vi "Save DAQ Configuration.vi"(8 "Error In":errorcluster, 10 "DAQ Device Settings":T1={"Analog Input Channel"="Dev1/ai0", "AImin[V]"=0, "AImax[V]"=5, "Analog Output Channel"="Dev1/ao0", "AOmin[V]"=0, "AOmax[V]"=5} {"AOmax[V]" min=-10 max=10 step=1 format="%.0g"; "AOmin[V]" min=-10 max=10 step=1 format="%.0g"; "AImax[V]" min=-10 max=10 step=1 format="%.0g"; "AImin[V]" min=-10 max=10 step=1 format="%.0g"}) -> (0 "Error Out":errorcluster)   [LabVIEW 2018]
uses:
  <vilib>/Utility/config.llb/Write Key (String).vi
  <vilib>/Utility/config.llb/Write Key (I32).vi
  <vilib>/Utility/config.llb/NI_LVConfig.lvlib
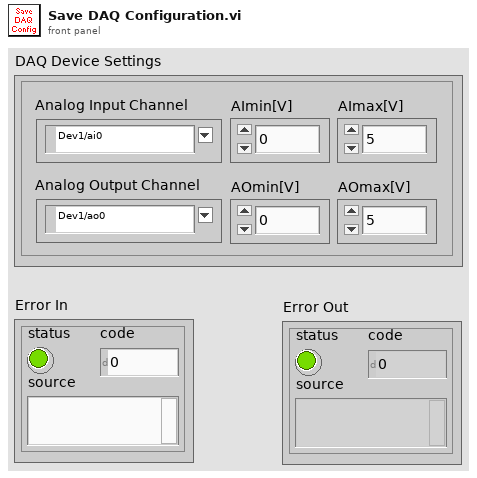
[diagram p1: front panel]
types:
  T1 = cluster{"Analog Input Channel":tag, "AImin[V]":i32, "AImax[V]":i32, "Analog Output Channel":tag, "AOmin[V]":i32, "AOmax[V]":i32}
  T2 = typedef "NI_LVConfig.lvlib/Config Data RefNum.ctl" = refnum<k1>
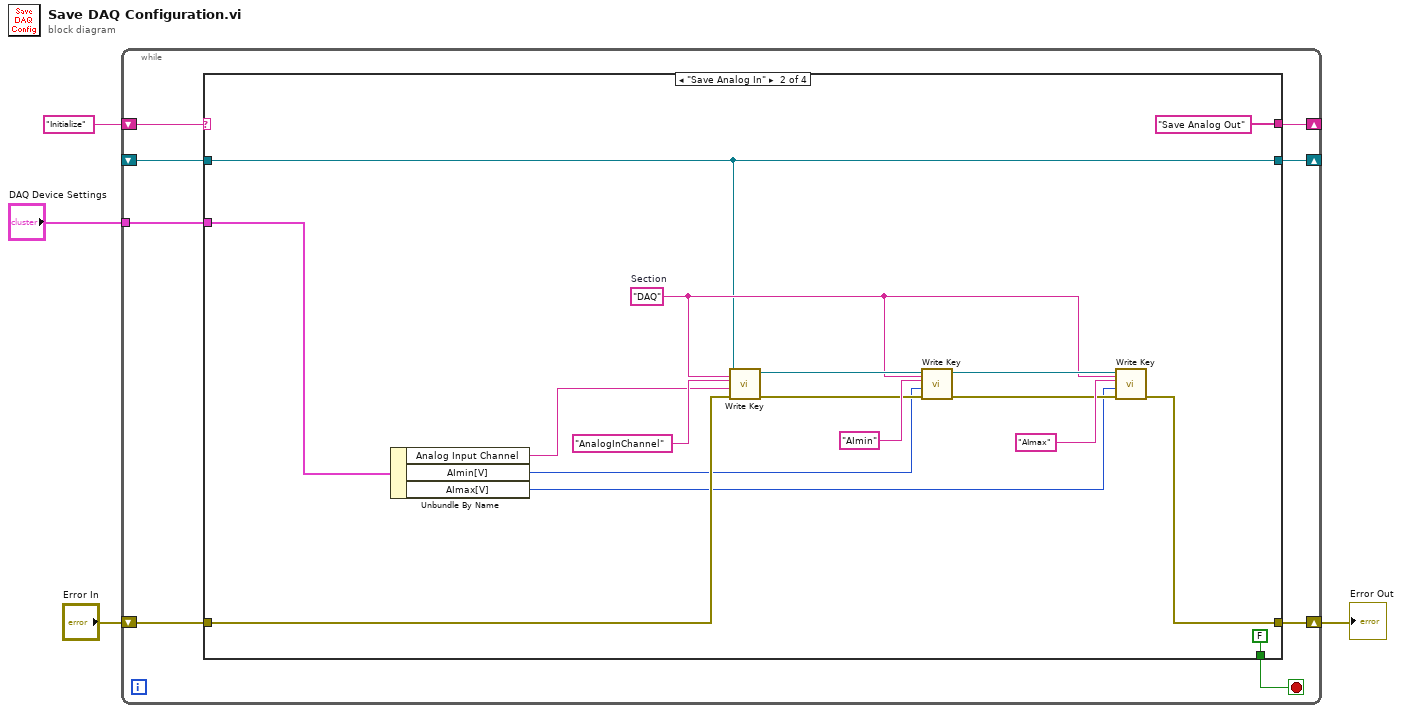
[diagram p0: block diagram]
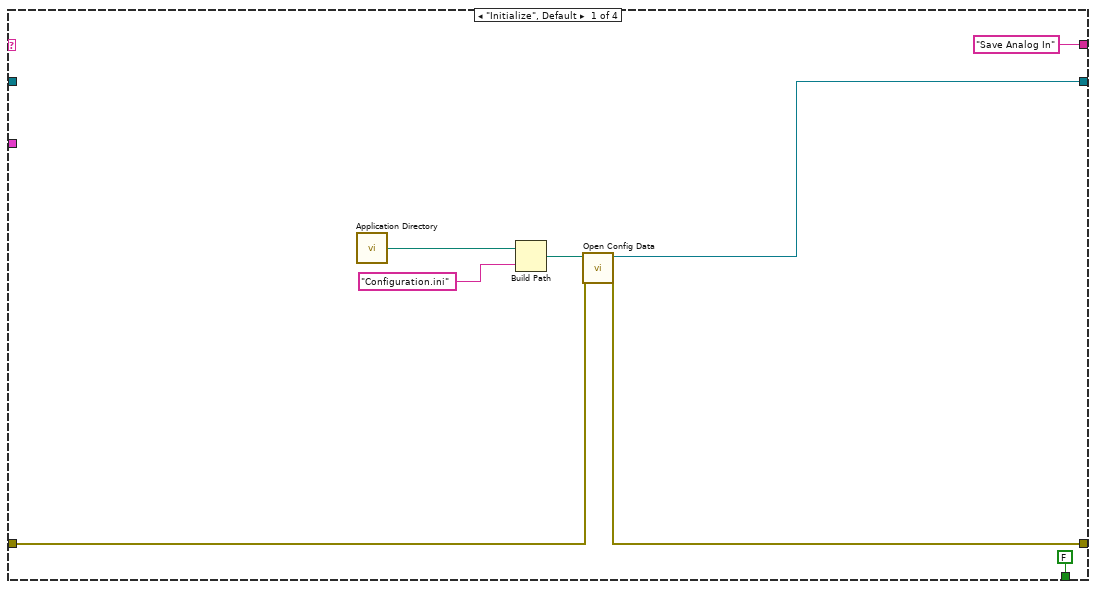
[diagram p2: hidden frame]
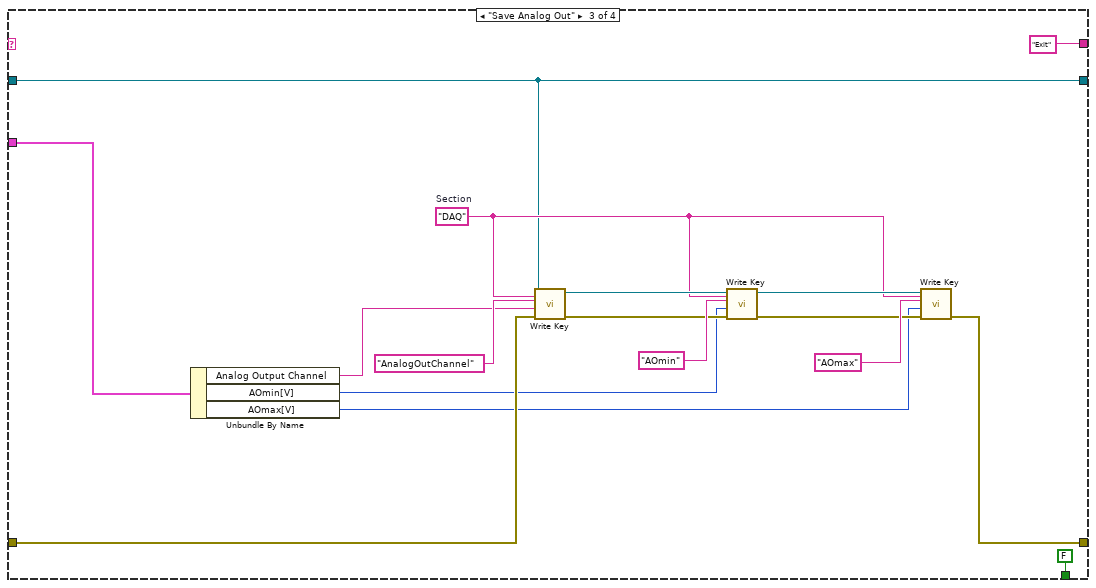
[diagram p3: hidden frame]
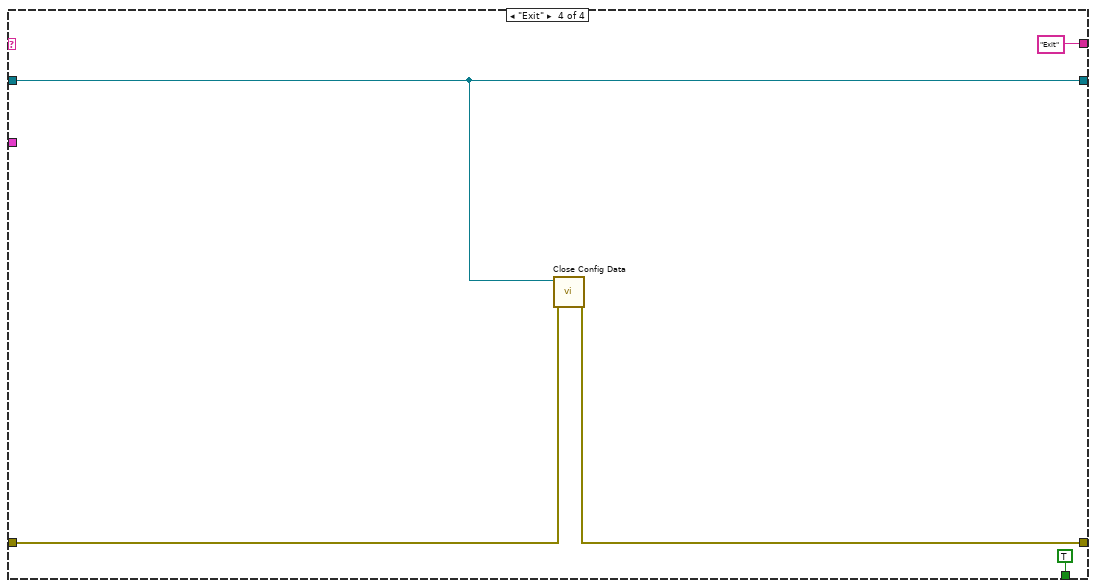
[diagram p4: hidden frame]
diagram:
  n1 = while {
    shift-right: [w8] -> _
    shift-left: "Initialize" ("key") -> [w12]
    shift-right: [w9] -> _
    shift-left: _ -> [w11]
    shift-right: [w6] -> w2
    shift-left: "Error In" -> [w10]
    tunnel: "DAQ Device Settings" -> [w5]
    stop <- w7 stop-if-true
    n2 = case shown="\"Save Analog In\"" w12 {
      tunnel: w11 -> [_ w23 w40 w57]
      tunnel: w10 -> [w14 w27 w44 w56]
      tunnel: [w15 w23 w40 w57] -> w9
      tunnel: ["Save Analog In" ("key") "Save Analog Out" ("key") "Exit" ("key") "Exit" ("key")] -> w8
      tunnel: [FALSE FALSE FALSE TRUE] -> w7
      tunnel: [w13 w21 w38 w55] -> w6
      tunnel: w5 -> [_ w22 w39 _]
      frame "Initialize", Default {
        n3 = call <vilib>:"Application Directory.vi"() -> ("Application Directory"=w18:path)
        n4 = Build Path(base path=w18, name or relative path="Configuration.ini") -> (appended path=w16:path)
        n5 = call <vilib>:"Open Config Data.vi"("error in (no error)"=w14, "configuration file path"=w16) -> ("error out"=w13:errorcluster, "refnum"=w15:T2)  [unwired: 7 in, 1 out]
      }
      frame "Save Analog In" {
        w28 = "DAQ"  # Section
        n6 = Unbundle By Name(w22) -> ("Analog Input Channel"=w26:tag, "AImin[V]"=w25:i32, "AImax[V]"=w24:i32)
        n7 = call-poly <vilib>:"Write Key.vi"("section"=w28, "error in (no error)"=w27, "value"=w26, "key"="AnalogInChannel", "refnum"=w23) -> ("error out"=w34:errorcluster, "refnum out"=w33:T2)  [unwired: 4 in, 1 out]
        n8 = call-poly <vilib>:"Write Key.vi"("section"=w28, "error in (no error)"=w34, "value"=w25, "key"="AImin", "refnum"=w33) -> ("error out"=w29:errorcluster, "refnum out"=w30:T2)  [unwired: 4 in, 1 out]
        n9 = call-poly <vilib>:"Write Key.vi"("section"=w28, "error in (no error)"=w29, "value"=w24, "key"="AImax", "refnum"=w30) -> ("error out"=w21:errorcluster)  [unwired: 4 in, 2 out]
      }
      frame "Save Analog Out" {
        w45 = "DAQ"  # Section
        n10 = Unbundle By Name(w39) -> ("Analog Output Channel"=w43:tag, "AOmin[V]"=w42:i32, "AOmax[V]"=w41:i32)
        n11 = call-poly <vilib>:"Write Key.vi"("section"=w45, "error in (no error)"=w44, "value"=w43, "key"="AnalogOutChannel", "refnum"=w40) -> ("error out"=w51:errorcluster, "refnum out"=w50:T2)  [unwired: 4 in, 1 out]
        n12 = call-poly <vilib>:"Write Key.vi"("section"=w45, "error in (no error)"=w51, "value"=w42, "key"="AOmin", "refnum"=w50) -> ("error out"=w46:errorcluster, "refnum out"=w47:T2)  [unwired: 4 in, 1 out]
        n13 = call-poly <vilib>:"Write Key.vi"("section"=w45, "error in (no error)"=w46, "value"=w41, "key"="AOmax", "refnum"=w47) -> ("error out"=w38:errorcluster)  [unwired: 4 in, 2 out]
      }
      frame "Exit" {
        n14 = call <vilib>:"Close Config Data.vi"("error in (no error)"=w56, "refnum"=w57) -> ("error out"=w55:errorcluster)  [unwired: 8 in, 1 out]
      }
    }
  }
  "Error Out" <- w2
